vi "DHE_PrepareExp_cleanup.vi"(8 "error in (no error)":errorcluster) -> (0 "error out":errorcluster)   [LabVIEW 2016]
uses:
  Common/public/vis/CMN_FVAR_action.ctl
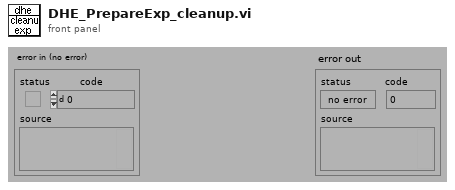
[diagram p1: front panel]
types:
  T1 = typedef "CMN_FVAR_action.ctl" = enum16{"read", "write"}
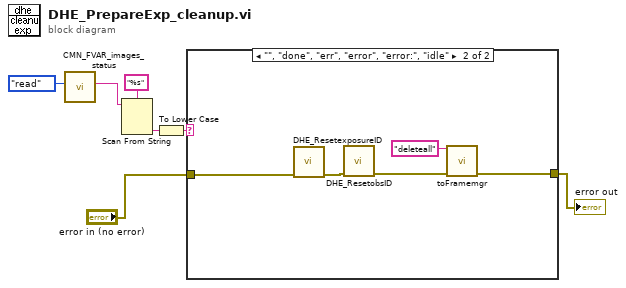
[diagram p0: block diagram]
diagram:
  n1 = call "CMN_FVAR_images_status.vi"("action"=CMN_FVAR_action."read") -> ("value out"=w4:string)  [unwired: 1 in, 8 out]
  n2 = Scan From String(format string="%s", input string=w4) -> (output 1=w2:string)  [unwired: 2 in, 4 out]
  n3 = To Lower Case(string=w2) -> (all lower case string=w1:string)
  n4 = case shown="\"\", \"done\", \"err\", \"error\", \"error:\", \"idle\"" w1 {
    tunnel: "error in (no error)" -> [w8 w10]
    tunnel: [w8 w9] -> w5
    frame Default {
    }
    frame "", "done", "err", "error", "error:", "idle" {
      n5 = call "DHE_ResetexposureID.vi"("error in (no error)"=w10) -> ("error out"=w13:errorcluster)  [unwired: 10 out]
      n6 = call "DHE_ResetobsID.vi"("error in (no error)"=w13) -> ("error out"=w11:errorcluster)  [unwired: 10 out]
      n7 = call "toFramemgr.vi"("command"="deleteall", "error in"=w11) -> ("error out"=w9:errorcluster)  [unwired: 7 in, 6 out]
    }
  }
  "error out" <- w5
